vi "csu.vi"() -> ()   [LabVIEW 2017]
panel:
  in  "stop":bool
  in  "close shutter":bool
  in  "open shutter":bool
  # "CSU"
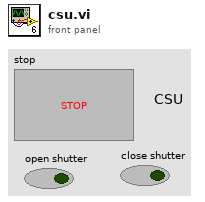
[diagram p1: front panel]
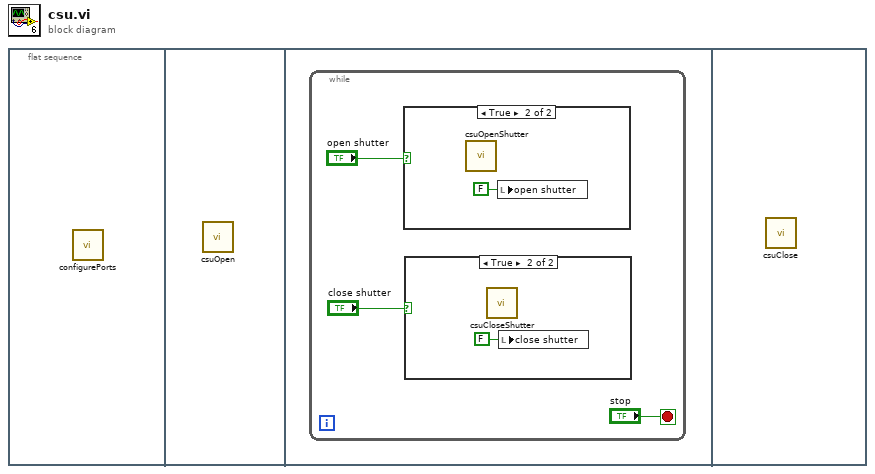
[diagram p0: block diagram]
diagram:
  n1 = flat-sequence {
    frame #0 {
      n2 = call "configurePorts.vi"() -> ()  [unwired: 12 in]
    }
    frame #1 {
      n3 = call "csuOpen.vi"() -> ()  [unwired: 14 in, 2 out]
    }
    frame #2 {
      n4 = while {
        stop <- "stop" stop-if-true
        n5 = case shown="True" "open shutter" {
          frame False {
          }
          frame True {
            n6 = call "csuOpenShutter.vi"() -> ()  [unwired: 16 in]
            n7 = local write "open shutter"(FALSE ("open shutter")) -> ()
          }
        }
        n8 = case shown="True" "close shutter" {
          frame False {
          }
          frame True {
            n9 = call "csuCloseShutter.vi"() -> ()  [unwired: 16 in]
            n10 = local write "close shutter"(FALSE ("open shutter")) -> ()
          }
        }
      }
    }
    frame #3 {
      n11 = call "csuClose.vi"() -> ()  [unwired: 12 in]
    }
  }
